vi "Auto Rotate Encoder.vi"(8 "error in (no error)":errorcluster, 10 "Rotation":dbl, 11 "Auto Refs":T2={"Ultrasonic Forward"={"AIDeviceRef"={"DevStatus"={"status"=FALSE, "code"=0, "source"=""}, "Controller"=enum."Controller 1", "Analog Channel"=enum."AI MXP 0"}, "Scaling factor (V/in)"=0.009585, "Average Bits"=3}, "Ultrasonic Back"={"AIDeviceRef"={"DevStatus"={"status"=FALSE, "code"=0, "source"=""}, "Controller"=enum."Controller 1", "Analog Channel"=enum."AI MXP 1"}, "Scaling factor (V/in)"=0.009585, "Average Bits"=3}, "Strafe Motor"={"DeviceStatus"={"status"=FALSE, "code"=0, "source"=""}, "Type"=enum."CANTalonSRX", "PWM"={"Controller"=enum."Controller 1", "PWM Channel"=enum."PWM 1", "DeadBand"={"Name"="", "maxPositivePwm"=0, "minPositivePwm"=0, "centerPwm"=0, "maxNegativePwm"=0, "minNegativePwm"=0, "angularRange"=0}}, "CAN"={"Device Number"=7, "Control Mode"=enum."Percent VBus", "Semaphore"=refnum, "Max Vout"=12.0, "TalonSRX Control Mode"=enum."Percent VBus"}, "Invert"=FALSE, "TransformRef"=refnum, "InvTransformRef"=refnum}, "Drive Motors"={"DevStatus"={"status"=FALSE, "code"=0, "source"=""}, "Motors[]"=[{"DeviceStatus"={"status"=FALSE, "code"=0, "source"=""}, "Type"=enum."CANTalonSRX", "PWM"={"Controller"=enum."Controller 1", "PWM Channel"=enum."PWM 1", "DeadBand"={"Name"="", "maxPositivePwm"=0, "minPositivePwm"=0, "centerPwm"=0, "maxNegativePwm"=0, "minNegativePwm"=0, "angularRange"=0}}, "CAN"={"Device Number"=4, "Control Mode"=enum."Percent VBus", "Semaphore"=refnum, "Max Vout"=12.0, "TalonSRX Control Mode"=enum."Percent VBus"}, "Invert"=FALSE, "TransformRef"=refnum, "InvTransformRef"=refnum}, {"DeviceStatus"={"status"=FALSE, "code"=0, "source"=""}, "Type"=enum."CANTalonSRX", "PWM"={"Controller"=enum."Controller 1", "PWM Channel"=enum."PWM 1", "DeadBand"={"Name"="", "maxPositivePwm"=0, "minPositivePwm"=0, "centerPwm"=0, "maxNegativePwm"=0, "minNegativePwm"=0, "angularRange"=0}}, "CAN"={"Device Number"=6, "Control Mode"=enum."Percent VBus", "Semaphore"=refnum, "Max Vout"=12.0, "TalonSRX Control Mode"=enum."Percent VBus"}, "Invert"=TRUE, "TransformRef"=refnum, "InvTransformRef"=refnum}, {"DeviceStatus"={"status"=FALSE, "code"=0, "source"=""}, "Type"=enum."CANTalonSRX", "PWM"={"Controller"=enum."Controller 1", "PWM Channel"=enum."PWM 1", "DeadBand"={"Name"="", "maxPositivePwm"=0, "minPositivePwm"=0, "centerPwm"=0, "maxNegativePwm"=0, "minNegativePwm"=0, "angularRange"=0}}, "CAN"={"Device Number"=3, "Control Mode"=enum."Percent VBus", "Semaphore"=refnum, "Max Vout"=12.0, "TalonSRX Control Mode"=enum."Percent VBus"}, "Invert"=FALSE, "TransformRef"=refnum, "InvTransformRef"=refnum}, {"DeviceStatus"={"status"=FALSE, "code"=0, "source"=""}, "Type"=enum."CANTalonSRX", "PWM"={"Controller"=enum."Controller 1", "PWM Channel"=enum."PWM 1", "DeadBand"={"Name"="", "maxPositivePwm"=0, "minPositivePwm"=0, "centerPwm"=0, "maxNegativePwm"=0, "minNegativePwm"=0, "angularRange"=0}}, "CAN"={"Device Number"=5, "Control Mode"=enum."Percent VBus", "Semaphore"=refnum, "Max Vout"=12.0, "TalonSRX Control Mode"=enum."Percent VBus"}, "Invert"=TRUE, "TransformRef"=refnum, "InvTransformRef"=refnum}], "Square Inputs"=TRUE, "Max Output"=1.0}, "Gyro"={"DevStatus"={"status"=FALSE, "code"=0, "source"=""}, "Analog Module"=enum."Controller 1", "Analog Channel"=enum."AI 0", "Offset"=0.0, "Gain (VoltsPerDegree/Second)"=0.007}} {"Ultrasonic Back"."Average Bits" max=15; "Ultrasonic Forward"."Average Bits" max=15}) -> (0 "error out":errorcluster)   [LabVIEW 2014]
uses:
  Auto Refs.ctl
  <vilib>/Rock Robotics/WPI/Ultrasonic/WPI_SonarMB1010AnalogDeviceRef.ctl
  <vilib>/Rock Robotics/WPI/AnalogChannel/WPI_AnalogChannelDevRef.ctl
  <vilib>/Rock Robotics/SystemInterfaces/Typedef/FPGA_TypedefAnalogModule.ctl
  <vilib>/Rock Robotics/SystemInterfaces/AI/FPGA_AIChannel.ctl
  <vilib>/Rock Robotics/WPI/MotorControl/WPI_MotorControlDeviceRef.ctl
  <vilib>/Rock Robotics/WPI/MotorControl/WPI_MotorControlType.ctl
  <vilib>/Rock Robotics/SystemInterfaces/Typedef/FPGA_TypedefDigitalModule.ctl
  <vilib>/Rock Robotics/SystemInterfaces/DIO/FPGA_DIOPWMChannel.ctl
  <vilib>/Rock Robotics/WPI/PWM/WPI_PWMDeadband.ctl
  <vilib>/Rock Robotics/WPI/CAN/Jaguar/SubVIs/WPI_CANJaguar_ControlMode.ctl
  <vilib>/Rock Robotics/WPI/CAN/TalonSRX/WPI_CANTalonSRX_APIControlMode.ctl
  <vilib>/Rock Robotics/WPI/PWM/WPI_PWMTransform_ConPane.ctl
  <vilib>/Rock Robotics/WPI/RobotDrive/WPI_RobotDriveDevRef.ctl
  <vilib>/Rock Robotics/WPI/Gyro/WPI_GyroDevRef.ctl
  Utilities/Refname.ctl
  Utilities/RefnameToString.vi
  <vilib>/Rock Robotics/WPI/RobotDrive/WPI_RobotDriveGetSetRefNum.vi
  <vilib>/addons/control/pid/pid.llb/PID (DBL).vi
  <vilib>/Rock Robotics/WPI/RobotDrive/WPI_RobotDriveArcadeDrive_Standard(NoSaturation).vi
  <vilib>/addons/control/pid/NI_PID_pid.lvlib
panel:
  in  "Rotation to encoder conversion":dbl
  in  "output range":cluster{"output high":dbl, "output low":dbl}={"output high"=0.85, "output low"=-0.85} {"output low" format="%.2f"; "output high" format="%.2f"}
  in  "PID gains":T1={"proportional gain (Kc)"=-0.0125, "integral time (Ti, min)"=0.025, "derivative time (Td, min)"=0.0} {"derivative time (Td, min)" format="%.3f"; "integral time (Ti, min)" format="%.3f"; "proportional gain (Kc)" min=-0.1 max=0.1 step=0.0001 format="%.6f"}
  in  "Feed Forward":dbl=0.19
  in  "Disable PID?":bool
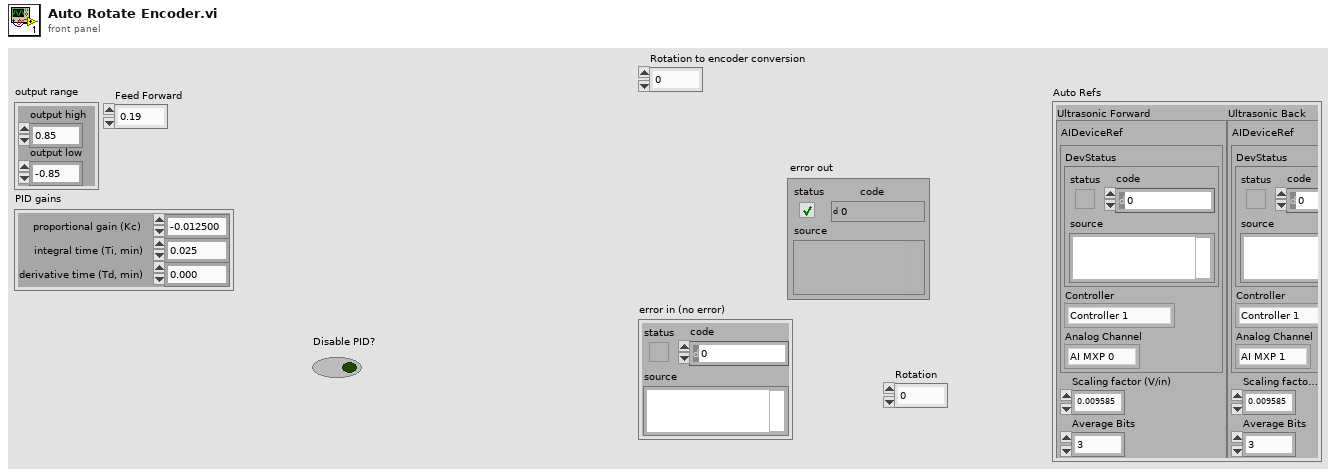
[diagram p1: front panel]
types:
  T1 = cluster{"proportional gain (Kc)":dbl, "integral time (Ti, min)":dbl, "derivative time (Td, min)":dbl}
  T2 = typedef "Auto Refs.ctl" = cluster{"Ultrasonic Forward":T3, "Ultrasonic Back":T3, "Strafe Motor":T7, "Drive Motors":T16, "Gyro":T17}
  T3 = typedef "WPI_SonarMB1010AnalogDeviceRef.ctl" = cluster{"AIDeviceRef":T4, "Scaling factor (V/in)":dbl, "Average Bits":u8}
  T4 = typedef "WPI_AnalogChannelDevRef.ctl" = cluster{"DevStatus":errorcluster, "Controller":T5, "Analog Channel":T6}
  T5 = typedef "FPGA_TypedefAnalogModule.ctl" = enum16{"Controller 1"}
  T6 = typedef "FPGA_AIChannel.ctl" = enum8{"AI 0", "AI 1", "AI 2", "AI 3", "AI MXP 0", "AI MXP 1", "AI MXP 2", "AI MXP 3", "Invalid"}
  T7 = typedef "WPI_MotorControlDeviceRef.ctl" = cluster{"DeviceStatus":errorcluster, "Type":T8, "PWM":cluster{"Controller":T9, "PWM Channel":T10, "DeadBand":T11}, "CAN":cluster{"Device Number":u8, "Control Mode":T12, "Semaphore":T13, "Max Vout":dbl, "TalonSRX Control Mode":T14}, "Invert":bool, "TransformRef":T15, "InvTransformRef":T15}
  T8 = typedef "WPI_MotorControlType.ctl" = enum16{"PWM", "CAN", "CANTalonSRX"}
  T9 = typedef "FPGA_TypedefDigitalModule.ctl" = enum16{"Controller 1"}
  T10 = typedef "FPGA_DIOPWMChannel.ctl" = enum8{"PWM 0", "PWM 1", "PWM 2", "PWM 3", "PWM 4", "PWM 5", "PWM 6", "PWM 7", "PWM 8", "PWM 9", "PWM MXP 0", "PWM MXP 1", "PWM MXP 2", "PWM MXP 3", "PWM MXP 4", "PWM MXP 5", "PWM MXP 6", "PWM MXP 7", "PWM MXP 8", "PWM MXP 9", "Invalid"}
  T11 = typedef "WPI_PWMDeadband.ctl" = cluster{"Name":string, "maxPositivePwm":i32, "minPositivePwm":i32, "centerPwm":i32, "maxNegativePwm":i32, "minNegativePwm":i32, "angularRange":u16}
  T12 = typedef "WPI_CANJaguar_ControlMode.ctl" = enum8{"Percent VBus", "Current", "Speed", "Position", "Voltage"}
  T13 = typedef "Semaphore RefNum" = refnum<k1>
  T14 = typedef "WPI_CANTalonSRX_APIControlMode.ctl" = enum8{"Percent VBus", "Speed", "Position", "Slave", "Unchanged / Invalid"}
  T15 = typedef "WPI_PWMTransform_ConPane.ctl" = refnum<vi>
  T16 = typedef "WPI_RobotDriveDevRef.ctl" = cluster{"DevStatus":errorcluster, "Motors[]":T7[], "Square Inputs":bool, "Max Output":dbl}
  T17 = typedef "WPI_GyroDevRef.ctl" = cluster{"DevStatus":errorcluster, "Analog Module":T5, "Analog Channel":T6, "Offset":dbl, "Gain (VoltsPerDegree/Second)":dbl}
  T18 = typedef "Refname.ctl" = enum16{"Gamepad 1", "Gamepad 2", "Drive Motors", "Strafe Motor", "Arm Clapper Motor", "Arm Angle", "Arm Belt Left", "Arm Belt Right", "Elevator 1", "Elevator 2", "Wiper"}
  T19 = typedef "WPI_CANTalonSRX_GlobalStatus.ctl" = cluster{"Applied Throttle":dbl, "Module Enabled":bool, "CAN Error":errorcluster, "Closed Loop Error":dbl, "Forward Limit Switch Closed":bool, "Reverse Limit Switch Closed":bool, "Sensor Position":dbl, "Sensor Velocity":dbl, "Current":dbl, "Sticky Fault - Over Temp":bool, "Sticky Fault - Under Voltage":bool, "Sticky Fault - Forward Limit":bool, "Sticky Fault - Reverse Limit":bool, "Sticky Fault - Forward Soft Limit":bool, "Sticky Fault - Reverse Soft Limit":bool, "Brake is Enabled":bool, "Encoder Position":dbl, "Encoder Velocity":dbl, "Encoder Index Count":dbl, "Encoder A Pin State":bool, "Encoder B Pin State":bool, "Encoder Index Pin State":bool, "Analog In":dbl, "Analog In Velocity":dbl, "Temperature (C)":dbl, "Battery Voltage":dbl}
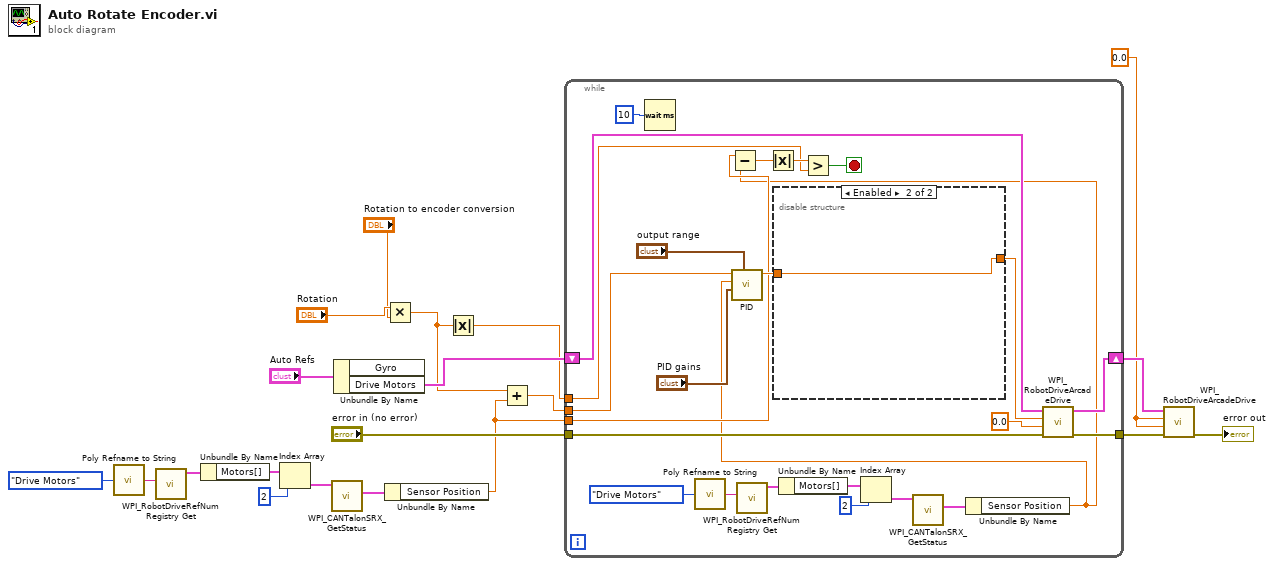
[diagram p0: block diagram]
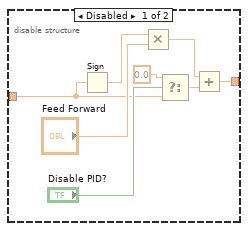
[diagram p2: hidden frame]
diagram:
  w16 = 0.0 ("X axis value")
  n1 = call-poly "Poly Refname to String.vi"("Enum"=Refname."Drive Motors") -> ("Refname"=w11:string)
  n2 = call <vilib>:"WPI_RobotDriveRefNum Registry Get.vi"("refnum name"=w11) -> ("RobotDriveDevRef"=w8:T16)  [unwired: 9 in, 1 out]
  n3 = Unbundle By Name(w8) -> ("Motors[]"=w9:T7[])
  n4 = Index Array(array=w9, index=2) -> (element=w7:T7)
  n5 = call <vilib>:"WPI_CANTalonSRX_GetStatus.vi"("CAN Talon SRX Ref"=w7) -> ("Talon SRX Status"=w6:T19)  [unwired: 8 in, 2 out]
  n6 = Unbundle By Name("Auto Refs") -> ("Drive Motors"=w19:T16)  [unwired: 1 out]
  n7 = Multiply(x="Rotation", y="Rotation to encoder conversion") -> (x*y=w3:dbl)
  n8 = Unbundle By Name(w6) -> ("Sensor Position"=w4:dbl)
  n9 = Absolute Value(x=w3) -> (abs(x)=w12:dbl)
  n10 = Add(x=w3, y=w4) -> (x+y=w20:dbl)
  n11 = while {
    tunnel: w20 -> [w35]
    tunnel: "error in (no error)" -> [w30]
    shift-right: [w39] -> w17
    shift-left: w19 -> [w40]
    tunnel: [w38] -> w18
    tunnel: w12 -> [w36]
    tunnel: w4 -> [w29]
    stop <- w31 stop-if-true
    n12 = Wait (ms)(milliseconds to wait=u32 10) -> ()  [unwired: 1 out]
    n13 = call-poly "Poly Refname to String.vi"("Enum"=Refname."Drive Motors") -> ("Refname"=w22:string)
    n14 = call <vilib>:"WPI_RobotDriveRefNum Registry Get.vi"("refnum name"=w22) -> ("RobotDriveDevRef"=w25:T16)  [unwired: 9 in, 1 out]
    n15 = Unbundle By Name(w25) -> ("Motors[]"=w24:T7[])
    n16 = Index Array(array=w24, index=2) -> (element=w26:T7)
    n17 = call <vilib>:"WPI_CANTalonSRX_GetStatus.vi"("CAN Talon SRX Ref"=w26) -> ("Talon SRX Status"=w27:T19)  [unwired: 8 in, 2 out]
    n18 = Unbundle By Name(w27) -> ("Sensor Position"=w21:dbl)
    n19 = Subtract(x=w29, y=w21) -> (x-y=w34:dbl)
    n20 = call-poly <vilib>:"PID.vi"("output range"="output range", "PID gains"="PID gains", "process variable"=w21, "setpoint"=w35) -> ("output"=w32:dbl)  [unwired: 6 in, 1 out]
    n21 = Absolute Value(x=w34) -> (abs(x)=w37:dbl)
    n22 = disable-structure shown="Enabled" {
      disable-tunnel: [w52 w53] -> w33
      disable-tunnel: w32 -> [w47 w53]
      frame Disabled {
        n23 = Sign(1:w47) -> (0:w50:dbl)
        n24 = Multiply(x=w50, y="Feed Forward") -> (x*y=w51:dbl)
        n25 = Select(t=0.0, s="Disable PID?", f=w47) -> (s? t:f=w45:dbl)
        n26 = Add(x=w51, y=w45) -> (x+y=w52:dbl)
      }
      frame Enabled {
      }
    }
    n27 = Greater?(x=w37, y=w36) -> (0:w31:bool)
    n28 = call-poly <vilib>:"WPI_RobotDriveArcadeDrive.vi"("error in (no error)"=w30, "Y axis value"=0.0, "X axis value"=w33, "RobotDriveDevRef"=w40) -> ("error out"=w38:errorcluster, "RobotDriveDevRef"=w39:T16)  [unwired: 5 in, 1 out]
  }
  n29 = call-poly <vilib>:"WPI_RobotDriveArcadeDrive.vi"("error in (no error)"=w18, "Y axis value"=w16, "X axis value"=w16, "RobotDriveDevRef"=w17) -> ("error out"=→"error out":errorcluster)  [unwired: 5 in, 2 out]
